vi "Write cam cluster.vi"(8 "error in (no error)":errorcluster, 10 "cam ref":T1, 11 "CameraSession in":refnum<class "CameraSession.lvclass">) -> (0 "error out":errorcluster, 3 "CameraSession out":refnum<class "CameraSession.lvclass">)   [LabVIEW 2013, in "CameraSession.lvclass"]
uses:
  CameraSession.lvclass
  SubVis/CamCluster.ctl
  <vilib>/vision/Image Controls.llb/IMAQ Image.ctl
  CameraSession.lvclass/CameraSession.ctl
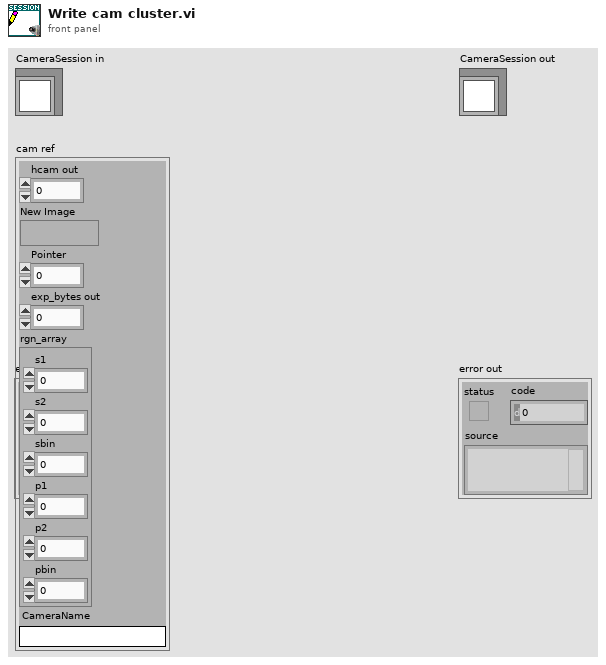
[diagram p1: front panel]
types:
  T1 = typedef "CamCluster.ctl" = cluster{"hcam out":i16, "New Image":T2, "Pointer":u32, "exp_bytes out":u32, "rgn_array":cluster{"s1":u16, "s2":u16, "sbin":u16, "p1":u16, "p2":u16, "pbin":u16}, "CameraName":string}
  T2 = typedef "IMAQ Image.ctl" = refnum<image>
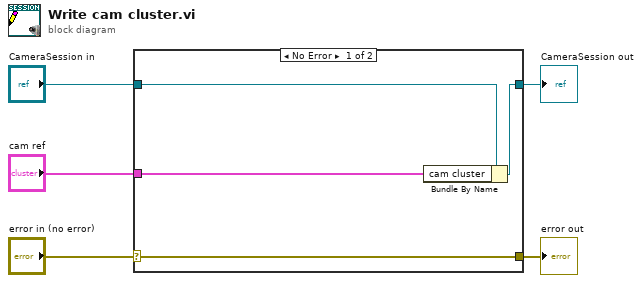
[diagram p0: block diagram]
diagram:
  n1 = case shown="No Error" "error in (no error)" {
    selector: "error in (no error)" -> [w9 w10]
    tunnel: [w9 w10] -> w4
    tunnel: [w7 w11] -> w2
    tunnel: "CameraSession in" -> [w8 w11]
    tunnel: "cam ref" -> [w6 _]
    frame No Error {
      n2 = Bundle By Name(cluster=w8, "cam cluster"=w6) -> (w7:refnum<class "CameraSession.lvclass">)
    }
    frame Error {
    }
  }
  "error out" <- w4
  "CameraSession out" <- w2
